vi "Gyro Global.vi"() -> ()   [LabVIEW 2013]
panel:
  in  "Names":string[](array[string])
  in  "Angle":dbl[](array[numeric])
  in  "Gain":dbl[](array[numeric])
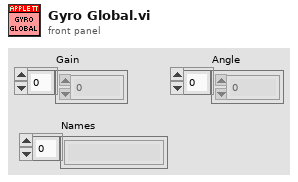
[diagram p1: front panel]
diagram:
